vi "Framework Main.vi"(8 "error in (no error)":errorcluster, 11 "Framework in":refnum<class "Framework.lvclass">) -> (0 "error out":errorcluster, 3 "Framework out":refnum<class "Framework.lvclass">)   [LabVIEW 2020]
uses:
  Includes/DSF Core.lvlibp/Classes/Framework/Framework.lvclass
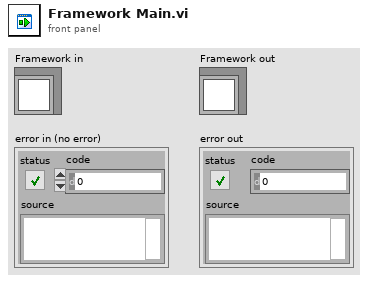
[diagram p1: front panel]
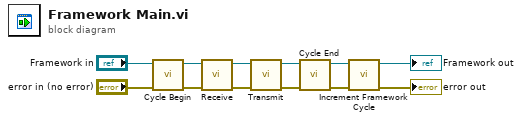
[diagram p0: block diagram]
diagram:
  n1 = call "Cycle Begin.vi"("error in (no error)"="error in (no error)", "Framework in"="Framework in") -> ("error out"=w5:errorcluster, "Framework out"=w6:refnum<class "Framework.lvclass">)  [unwired: 8 in]
  n2 = call "Receive.vi"("error in"=w5, "framework in"=w6) -> ("error out"=w12:errorcluster, "framework out"=w11:refnum<class "Framework.lvclass">)  [unwired: 8 in]
  n3 = call "Transmit.vi"("error in"=w12, "framework in"=w11) -> ("error out"=w3:errorcluster, "framework out"=w4:refnum<class "Framework.lvclass">)  [unwired: 8 in]
  n4 = call "Cycle End.vi"("error in (no error)"=w3, "Framework in"=w4) -> ("error out"=w1:errorcluster, "Framework out"=w2:refnum<class "Framework.lvclass">)  [unwired: 8 in]
  n5 = call "Increment Framework Cycle.vi"("error in (no error)"=w1, "Framework in"=w2) -> ("error out"=→"error out":errorcluster, "Framework out"=→"Framework out":refnum<class "Framework.lvclass">)  [unwired: 8 in]
